vi "ADIS16448_RoboRIO_Teensy_RefNum Registry Set.vi"(8 "error in (no error)":errorcluster, 10 "refnum name":string, 11 "SerialPortRef":T1) -> (0 "error out":errorcluster, 3 "SerialPortRefOut":T1)   [LabVIEW 2016, in "RoboRIO-Teensy-ADIS16448-Interface.lvlib"]
uses:
  <vilib>/Rock Robotics/WPI/SerialPort/WPI_SerialPortRef.ctl
  RoboRIO-Teensy-ADIS16448-Interface.lvlib
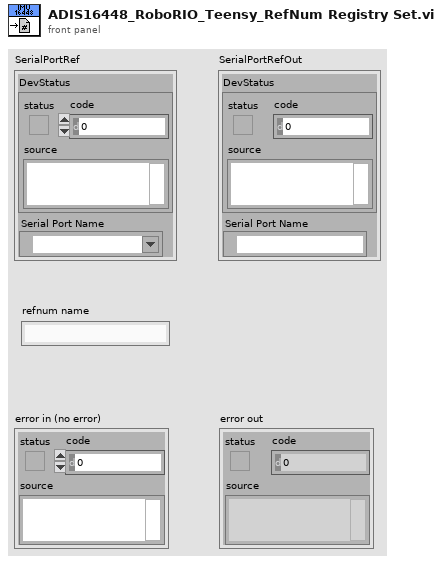
[diagram p1: front panel]
types:
  T1 = typedef "WPI_SerialPortRef.ctl" = cluster{"DevStatus":errorcluster, "Serial Port Name":refnum<visa-resource-name>}
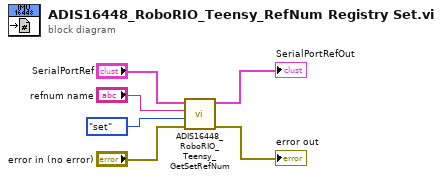
[diagram p0: block diagram]
diagram:
  n1 = call "ADIS16448_RoboRIO_Teensy_GetSetRefNum.vi"("error in (no error)"="error in (no error)", "menu"=enum16{"set", "get"}."set", "refnum name"="refnum name", "SerialPortRef"="SerialPortRef") -> ("error out"=→"error out":errorcluster, "SerialPortRefOut"=→"SerialPortRefOut":T1)  [unwired: 6 in]
